vi "Date and Shift Gen.vi"(10 "Error In":errorcluster) -> (2 "Error Out":errorcluster, 3 "DATE And SHIFT":string, 5 "MFG Date for SQL":string)   [LabVIEW 2018]
panel:
  # "DATE and SHIFT Generate"
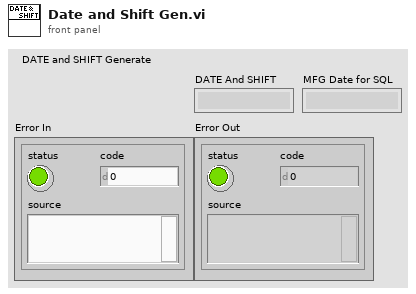
[diagram p1: front panel]
types:
  T1 = typedef "LVDateTimeRec.ctl" = cluster{"fractional second":dbl, "second":i32, "minute":i32, "hour":i32, "day of month":i32, "month":i32, "year":i32, "day of week":i32, "day of year":i32, "DST":i32}
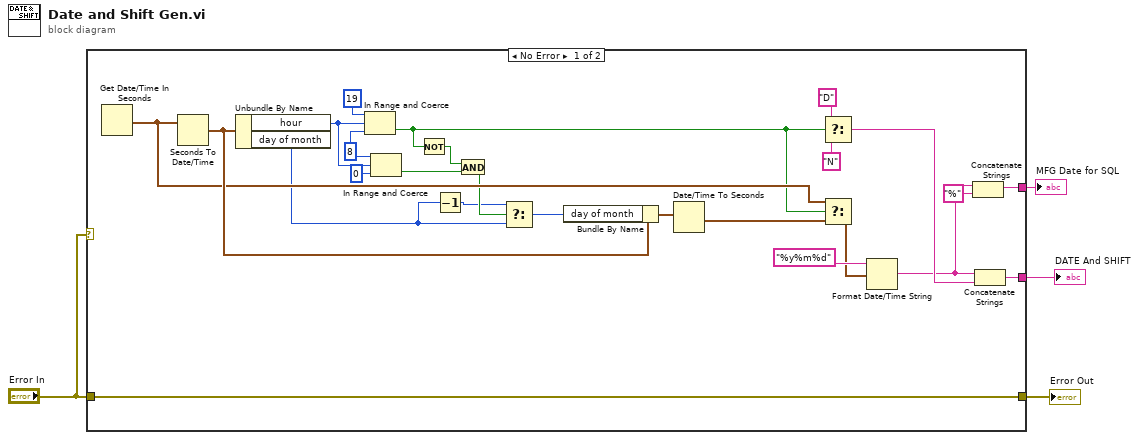
[diagram p0: block diagram]
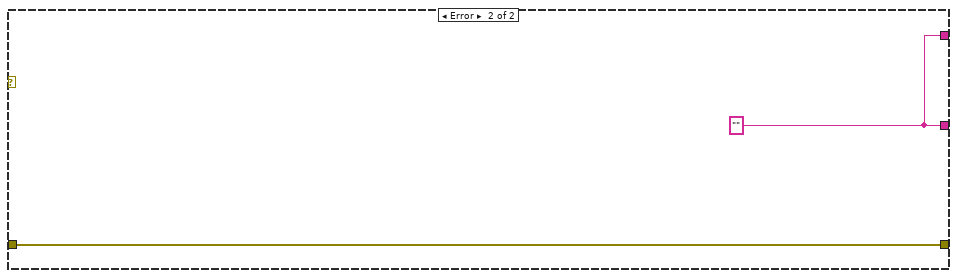
[diagram p2: hidden frame]
diagram:
  n1 = case shown="No Error" "Error In" {
    tunnel: [w19 w30] -> w4
    tunnel: "Error In" -> [w18 w31]
    tunnel: [w18 w31] -> w2
    tunnel: [w15 w30] -> w1
    frame No Error {
      w14 = i16 8 ("upper limit")
      n2 = Get Date/Time In Seconds() -> (seconds since 1Jan1904=w21:timestamp)
      n3 = Seconds To Date/Time(time stamp (now)=w21) -> (date time rec=w22:T1)  [unwired: 1 in]
      n4 = Unbundle By Name(w22) -> ("hour"=w5:i32, "day of month"=w7:i32)
      n5 = In Range and Coerce(upper limit=i16 19, x=w5, lower limit=w14) -> (In Range?=w10:bool)  [unwired: 1 out]
      n6 = In Range and Coerce(upper limit=w14, x=w5, lower limit=i16 0) -> (In Range?=w12:bool)  [unwired: 1 out]
      n7 = Not(x=w10) -> (.not. x?=w11:bool)
      n8 = Decrement(x=w7) -> (x-1=w8:i32)
      n9 = And(x=w11, y=w12) -> (x .and. y?=w9:bool)
      n10 = Select(t=w8, s=w9, f=w7) -> (s? t:f=w6:i32)
      n11 = Bundle By Name(cluster=w22, "day of month"=w6) -> (w25:T1)
      n12 = Date/Time To Seconds(2:w25) -> (0:w24:timestamp)  [unwired: 1 in]
      n13 = Select(t="D", s=w10, f="N") -> (s? t:f=w20:string)
      n14 = Select(t=w21, s=w10, f=w24) -> (s? t:f=w23:timestamp)
      n15 = Format Date/Time String(time format string (%c)="%y%m%d", seconds (now)=w23) -> (date/time string=w17:string)  [unwired: 1 in]
      n16 = Concatenate Strings(w17, "%" ("string")) -> (w15:string)
      n17 = Concatenate Strings(w17, w20) -> (w19:string)
    }
    frame Error {
      w30 = ""
    }
  }
  "Error Out" <- w2
  "DATE And SHIFT" <- w4
  "MFG Date for SQL" <- w1
